vi "unpack_object.vi"(3 "error in":errorcluster, 5 "u":u64) -> (0 "error out":errorcluster, 1 "var":variant, 2 "u out":u64)   [LabVIEW 2019, in "msgunpack.lvlib"]
doc: "Unpacks an object from the buffer stream and returns it as a variant. Complimentary to the pack_item VI\n\nSupported types are:\n- Numeric types\n- Arrays\n- Booleans\n- Strings (raw)\n- Attribute variants (map)\n- Null"
uses:
  msgunpack.lvlib
panel:
  # "msgpack"
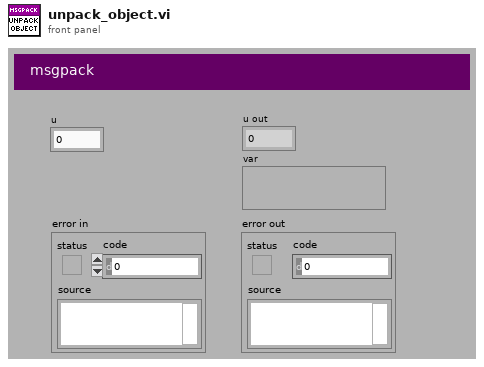
[diagram p1: front panel]
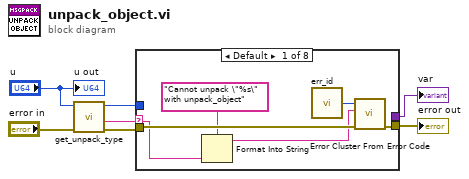
[diagram p0: block diagram]
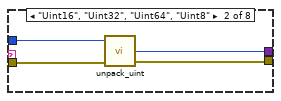
[diagram p2: hidden frame]
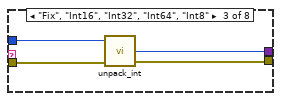
[diagram p3: hidden frame]
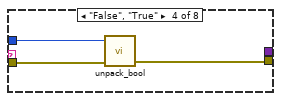
[diagram p4: hidden frame]
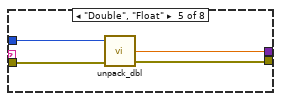
[diagram p5: hidden frame]
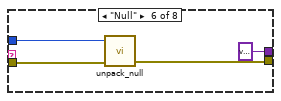
[diagram p6: hidden frame]
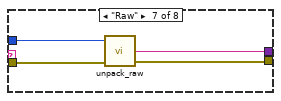
[diagram p7: hidden frame]
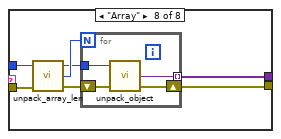
[diagram p8: hidden frame]
diagram:
  n1 = call "get_unpack_type.vi"("error in"="error in", "u"="u") -> ("error out"=w5:errorcluster, "name"=w4:string, "u out"=w3:u64)  [unwired: 2 in, 1 out]
  n2 = case shown="Default" w4 {
    selector: w4 -> [w11 _ _ _ _ _ _ _]
    tunnel: w5 -> [w12 w16 w20 w23 w27 w31 w35 w42]
    tunnel: w3 -> [_ w17 w21 w24 w28 w32 w36 w43]
    tunnel: [w13 w15 w19 w22 w26 w30 w34 w37] -> w2
    tunnel: [_ w14 w18 _ w25 variant w33 w38] -> w1
    frame Default {
      n3 = Format Into String(format string="Cannot unpack \"%s\" with unpack_object", w11) -> (resulting string=w10:string)  [unwired: 2 in, 1 out]
      n4 = call "err_id.vi"() -> ("error code"=w8:i32)
      n5 = call <vilib>:"Error Cluster From Error Code.vi"("error in (no error)"=w12, "error message (\"\")"=w10, "error code (0)"=w8) -> ("error out"=w13:errorcluster)  [unwired: 6 in]
    }
    frame "Uint16", "Uint32", "Uint64", "Uint8" {
      n6 = call "unpack_uint.vi"("error in"=w16, "u"=w17) -> ("error out"=w15:errorcluster, "uint64"=w14:u64)  [unwired: 1 in, 1 out]
    }
    frame "Fix", "Int16", "Int32", "Int64", "Int8" {
      n7 = call "unpack_int.vi"("error in"=w20, "u"=w21) -> ("error out"=w19:errorcluster, "int64"=w18:i64)  [unwired: 1 in, 1 out]
    }
    frame "False", "True" {
      n8 = call "unpack_bool.vi"("error in"=w23, "u"=w24) -> ("error out"=w22:errorcluster)  [unwired: 1 in, 2 out]
    }
    frame "Double", "Float" {
      n9 = call "unpack_dbl.vi"("error in"=w27, "u"=w28) -> ("error out"=w26:errorcluster, "dbl"=w25:dbl)  [unwired: 1 in, 1 out]
    }
    frame "Null" {
      n10 = call "unpack_null.vi"("error in"=w31, "u"=w32) -> ("error out"=w30:errorcluster)  [unwired: 2 in, 1 out]
    }
    frame "Raw" {
      n11 = call "unpack_raw.vi"("error in"=w35, "u"=w36) -> ("error out"=w34:errorcluster, "raw"=w33:string)  [unwired: 1 in, 1 out]
    }
    frame "Array" {
      n12 = call "unpack_array_len.vi"("error in"=w42, "u"=w43) -> ("error out"=w39:errorcluster, "n"=w41:u32, "u out"=w40:u64)  [unwired: 1 in]
      n13 = for {
        N: w41 -> [_]
        tunnel: w40 -> [w45]
        tunnel: [w44] -> w38 mode=indexing
        shift-right: [w46] -> w37
        shift-left: w39 -> [w47]
        n14 = call "unpack_object.vi"("error in"=w47, "u"=w45) -> ("error out"=w46:errorcluster, "var"=w44:variant)  [unwired: 1 in, 1 out]
      }
    }
  }
  "error out" <- w2
  "var" <- w1
  "u out" <- "u"
